vi "LV SCISDK Set Parameter U Integer.vi"(8 "error in (no error)":errorcluster, 9 "handle":u64, 10 "value":u32, 11 "Path":string) -> (0 "error out":errorcluster, 1 "handle out":u64, 3 "function return":i32)   [LabVIEW 2021, in "SciSDK_Labview.lvlib"]
doc: "SCISDKLABVIEW_DLL_API int LV_SCISDK_SetParameterUInteger(char* Path, unsigned int value, void* handle);"
uses:
  SciSDK_Labview.lvlib
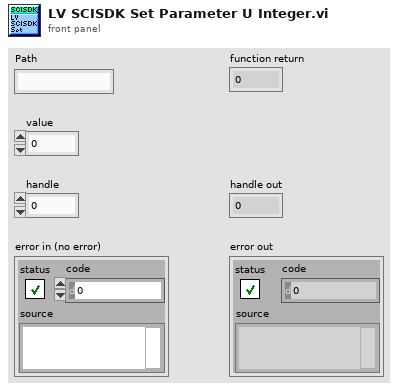
[diagram p1: front panel]
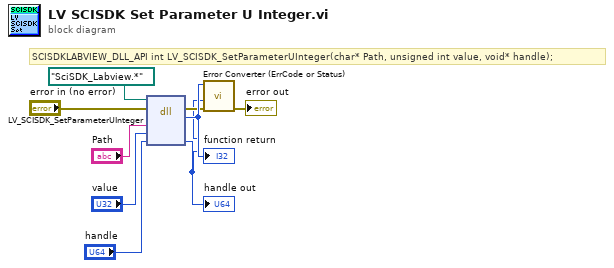
[diagram p0: block diagram]
diagram:
  # "SCISDKLABVIEW_DLL_API int LV_SCISDK_SetParameterUInteger(char* Path, unsigned int value, void* handle);"
  n1 = dll-call lib="C:/git/scisdk/SciSDK_VC++/x64/Debug/SciSDK_Labview.*" fn="LV_SCISDK_SetParameterUInteger"(path in=path "SciSDK_Labview.*", error in="error in (no error)", "Path"="Path", "value"="value", "handle"="handle") -> (error out=w4:errorcluster, "return type"=w9:i32, "handle"=w1:u64)  [unwired: 3 in, 1 out]
  "function return" <- w9
  "handle out" <- w1
  n2 = call "Error Converter (ErrCode or Status).vi"("error in (no error)"=w4, "handle"=w1, "error code"=w9) -> ("error out"=→"error out":errorcluster)  [unwired: 8 in]
